vi "Log Save to File LaunchPad.vi"(8 "data":dbl, 9 "datastream ID":i32, 10 "cycle":i32, 11 "filename":string="C:\\LILP_log.txt") -> ()   [LabVIEW 2010]
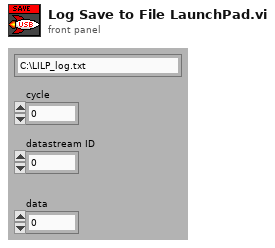
[diagram p1: front panel]
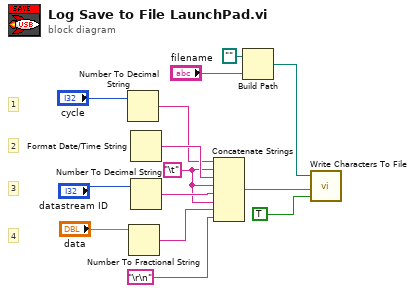
[diagram p0: block diagram]
diagram:
  w1 = "\t"
  # "4"
  # "3"
  # "2"
  # "1"
  n1 = Number To Decimal String(number="cycle") -> (decimal integer string=w6:string)  [unwired: 1 in]
  n2 = Number To Fractional String(number="data") -> (F-format string=w4:string)  [unwired: 3 in]
  n3 = Format Date/Time String ("Date/Time")() -> (date/time string=w8:string)  [unwired: 3 in]
  n4 = Number To Decimal String(number="datastream ID") -> (decimal integer string=w2:string)  [unwired: 1 in]
  n5 = Concatenate Strings(w6, w1, w8, w1, w2, w1, w4, "\r\n") -> (w10:string)
  n6 = Build Path(base path=path "", name or relative path="filename") -> (appended path=w13:path)
  n7 = call <vilib>:"Write Characters To File.vi"("append to file? (new file:F)"=TRUE, "character string"=w10, "file path (dialog if empty)"=w13) -> ()  [unwired: 3 out]
